vi "ABR3-Options Dialog.vi"(0 "Hidden":T2={"AO Samp Rate Hz"=0.0, "Duration (ms)"=100000.0, "Ramp (ms)"=5.0, "Click width (us)"=0.5}, 2 "Parent VI":refnum<vi>, 5 "Threshold Estimation In":T1) -> (4 "Cluster out":T2={"AO Samp Rate Hz"=0.0, "Duration (ms)"=100000.0, "Ramp (ms)"=5.0, "Click width (us)"=0.5}, 6 "Threshold Estimation Out":T1, 8 "Canceled?":bool)   [LabVIEW 2020]
uses:
  TypeDefs/ABR3-Hidden Params.ctl
  Threshold Estimation VIs/ABR3-Threshold Estimation Parameters.ctl
panel:
  in  "R2 criterion":dbl caption="Adj R2 criterion"
  in  "CC criterion":dbl caption="Corrcoef criterion"
  in  "Thr Tmax":dbl caption="Tmax (ms)"
  in  "Thr Tmin":dbl caption="Tmin (ms)"
  in  "ClickWidth":dbl caption="Click duration (us)"
  in  "ToneRamp":dbl caption="Tone burst ramp length (ms)"
  in  "ToneDur":dbl caption="Tone burst duration (ms)"
  in  "AO Fs":dbl caption="Output sampling rate (Hz)"
  in  "Cancel":bool
  in  "OK":bool
  # "Threshold estimation"
  # "Warning! Unless you're sure you know what you're doing, don't change these parameters"
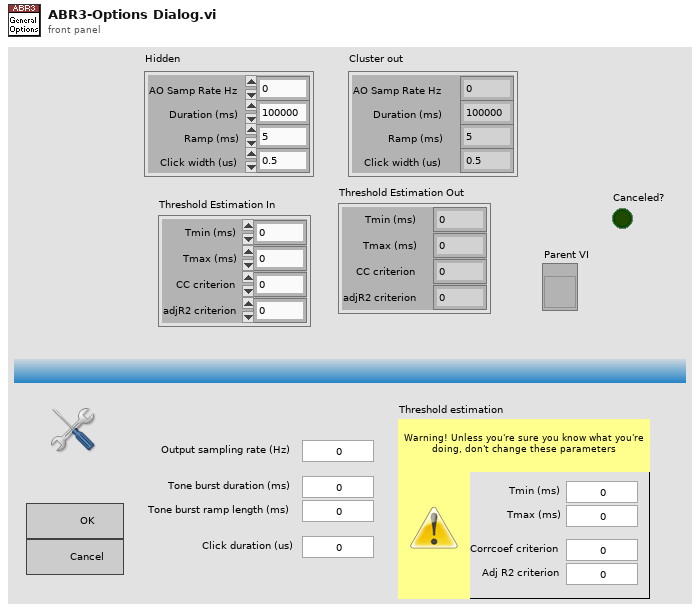
[diagram p1: front panel]
types:
  T1 = typedef "ABR3-Threshold Estimation Parameters.ctl" = cluster{"Tmin (ms)":dbl, "Tmax (ms)":dbl, "CC criterion":dbl, "adjR2 criterion":dbl}
  T2 = typedef "ABR3-Hidden Params.ctl" = cluster{"AO Samp Rate Hz":dbl, "Duration (ms)":dbl, "Ramp (ms)":dbl, "Click width (us)":dbl}
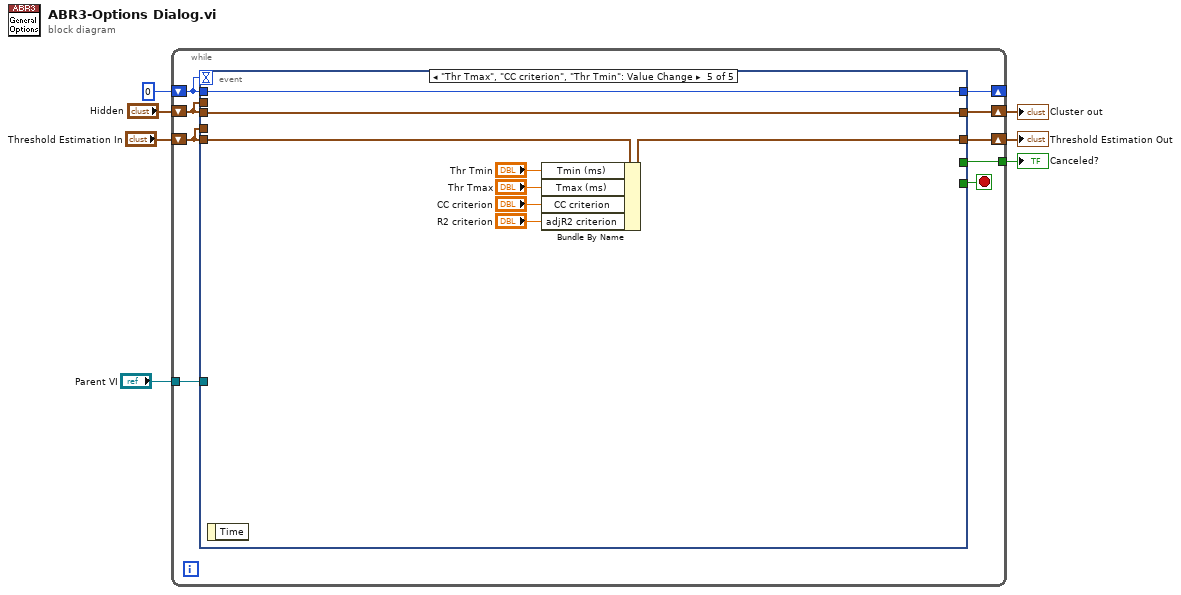
[diagram p0: block diagram]
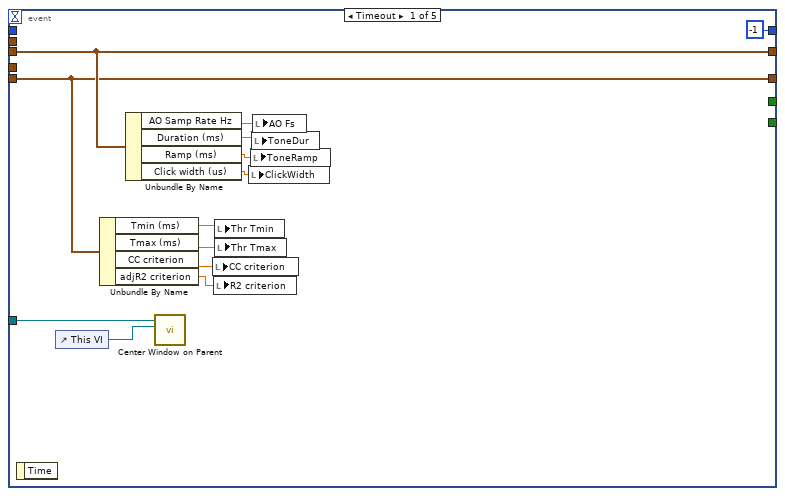
[diagram p2: hidden frame]
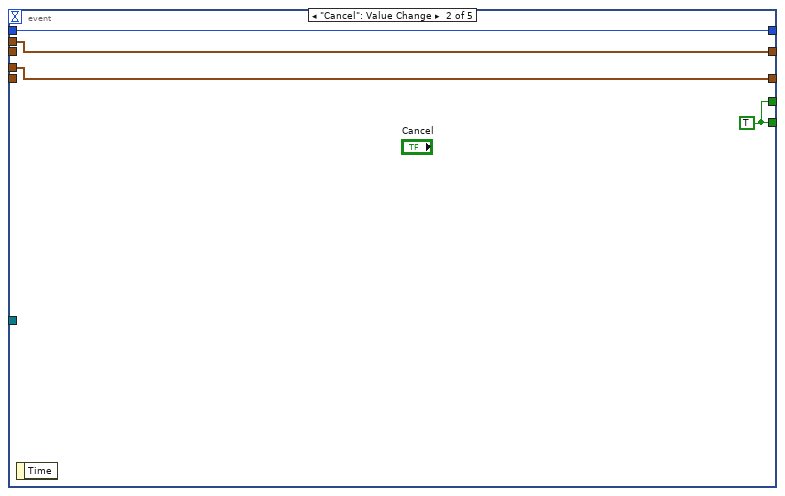
[diagram p3: hidden frame]
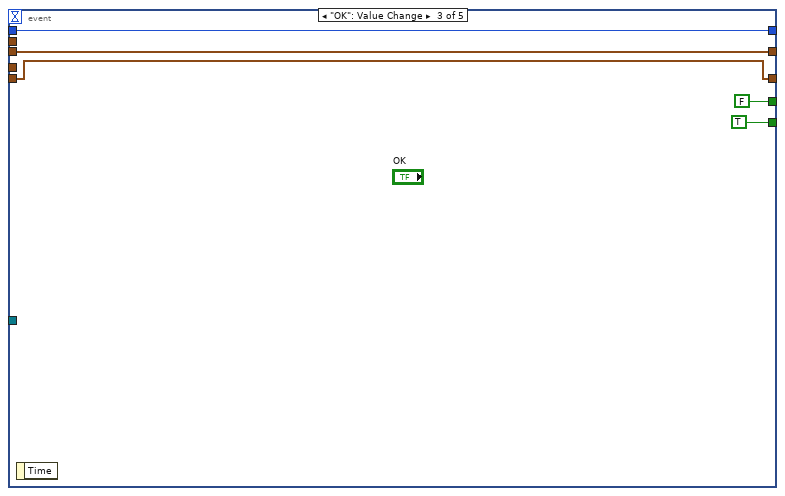
[diagram p4: hidden frame]
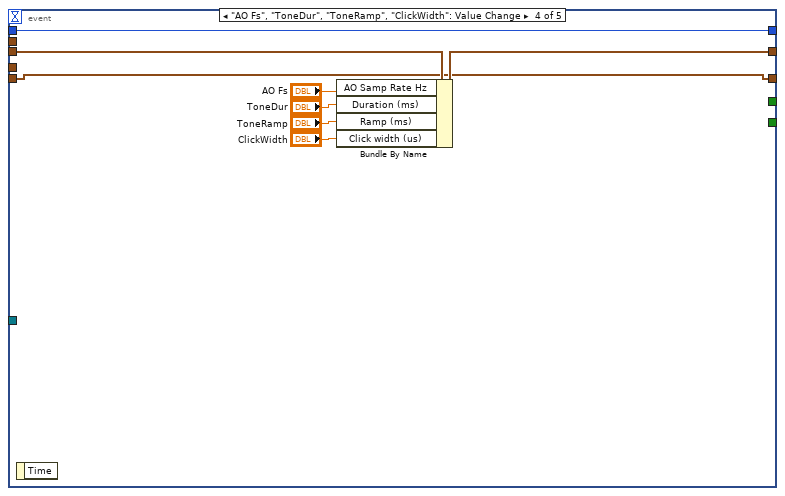
[diagram p5: hidden frame]
diagram:
  n1 = while {
    shift-right: [w16] -> _
    shift-left: 0 -> [w9]
    tunnel: [w13] -> w4
    shift-right: [w15] -> w5
    shift-left: "Hidden" -> [w12]
    shift-right: [w11] -> w2
    shift-left: "Threshold Estimation In" -> [w10]
    tunnel: "Parent VI" -> [w8]
    stop <- w14 stop-if-true
    n2 = event shown="[4] \"Thr Tmax\", \"CC criterion\", \"Thr Tmin\": Value Change" {
      selector: _ -> [_ _ _ _ _]
      dyn-events: _ -> [_ _ _ _ _]
      timeout: w9 -> [_ _ _ _ _]
      tunnel: [-1 w30 w34 w39 w50] -> w16
      tunnel: w12 -> [w28 _ w38 w46 w54]
      tunnel: [w28 w32 w38 w45 w54] -> w15
      tunnel: [_ w33 TRUE _ _] -> w14
      tunnel: [_ w33 FALSE _ _] -> w13
      tunnel: w12 -> [_ w32 _ _ _]
      tunnel: w10 -> [w23 _ w35 w40 w48]
      tunnel: [w23 w31 w35 w40 w47] -> w11
      tunnel: w10 -> [_ w31 _ _ _]
      tunnel: w9 -> [_ w30 w34 w39 w50]
      tunnel: w8 -> [w19 _ _ _ _]
      event Timeout {
        n3 = event-data() -> ()  [unwired: 1 in, 1 out]
        n4 = control-ref of="This VI"() -> (w18:refnum<vi>)
        n5 = Unbundle By Name(w23) -> ("Tmin (ms)"=w22:dbl, "Tmax (ms)"=w21:dbl, "CC criterion"=w20:dbl, "adjR2 criterion"=w17:dbl)
        n6 = Unbundle By Name(w28) -> ("AO Samp Rate Hz"=w27:dbl, "Duration (ms)"=w26:dbl, "Ramp (ms)"=w25:dbl, "Click width (us)"=w24:dbl)
        n7 = call "Center Window on Parent.vi"("Parent VI"=w18, "VI in"=w19) -> ()  [unwired: 8 in, 2 out]
        n8 = local write "CC criterion"(w20) -> ()
        n9 = local write "R2 criterion"(w17) -> ()
        n10 = local write "Thr Tmin"(w22) -> ()
        n11 = local write "Thr Tmax"(w21) -> ()
        n12 = local write "ClickWidth"(w24) -> ()
        n13 = local write "ToneRamp"(w25) -> ()
        n14 = local write "ToneDur"(w26) -> ()
        n15 = local write "AO Fs"(w27) -> ()
      }
      event "Cancel": Value Change {
        w33 = TRUE
        n16 = event-data() -> ()  [unwired: 1 in, 1 out]
      }
      event "OK": Value Change {
        n17 = event-data() -> ()  [unwired: 1 in, 1 out]
      }
      event "AO Fs", "ToneDur", "ToneRamp", "ClickWidth": Value Change {
        n18 = event-data() -> ()  [unwired: 1 in, 1 out]
        n19 = Bundle By Name(cluster=w46, "AO Samp Rate Hz"="AO Fs", "Duration (ms)"="ToneDur", "Ramp (ms)"="ToneRamp", "Click width (us)"="ClickWidth") -> (w45:T2)
      }
      event "Thr Tmax", "CC criterion", "Thr Tmin": Value Change {
        n20 = event-data() -> ()  [unwired: 1 in, 1 out]
        n21 = Bundle By Name(cluster=w48, "Tmin (ms)"="Thr Tmin", "Tmax (ms)"="Thr Tmax", "CC criterion"="CC criterion", "adjR2 criterion"="R2 criterion") -> (w47:T1)
      }
    }
  }
  "Cluster out" <- w5
  "Canceled?" <- w4
  "Threshold Estimation Out" <- w2
